vi "temp_till_try_and_error.vi"(6 "Timeout (10000 ms)":u32=10000, 8 "error in (no error)":errorcluster, 9 "Points":i32=250, 10 "Source Channel (0: Channel 1)":i32(ring) items=["Channel 1"=0, "Channel 2"=1, "Channel 3"=2, "Channel 4"=3, "Waveform Memory 1"=5, "Waveform Memory 2"=6, "Serial Bus 1"=7, "Serial Bus 2"=8, "Digital Bus Low"=9, "Digital Bus High "=10, "Digital Bus 1"=11, "Digital Bus 2"=12, "Function 1"=32, "Function 2"=33, "Function 3"=34, "Function 4"=35, "Math 1"=36, "Math 2"=37, "Math 3"=38, "Math 4"=39], 11 "VISA resource name":refnum<visa-resource-name>) -> (0 "error out":errorcluster, 2 "Waveform Data":waveform(dbl)[](graph), 3 "VISA resource name out":refnum<visa-resource-name>)   [LabVIEW 2016]
uses:
  <instrlib>/Agilent 2000 3000 X-Series/Agilent 2000 3000 X-Series.lvlib
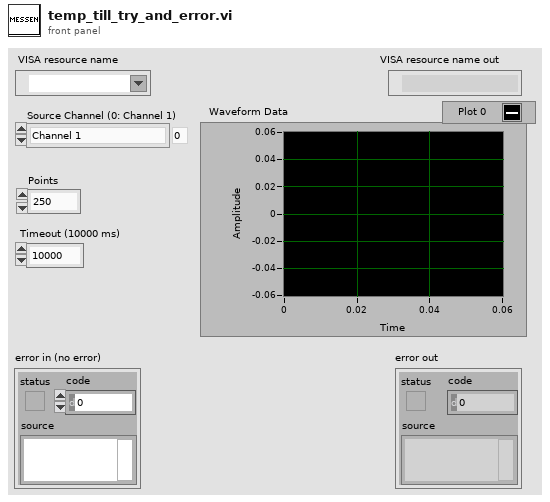
[diagram p1: front panel]
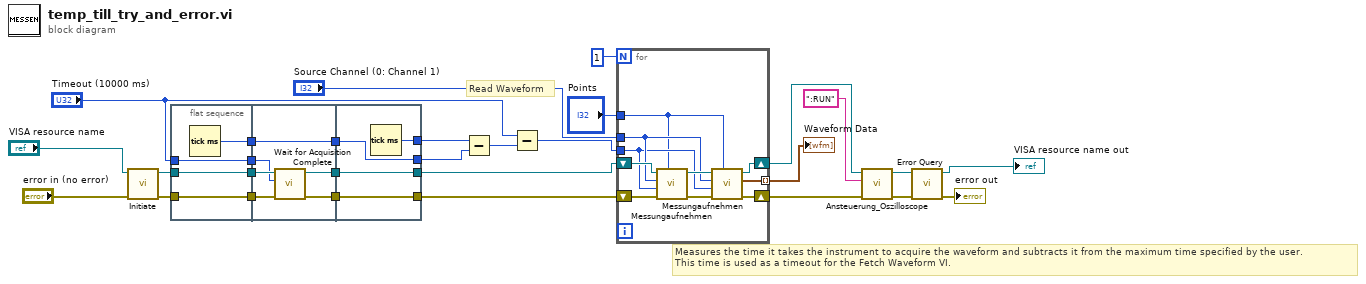
[diagram p0: block diagram]
diagram:
  # "Measures the time it takes the instrument to acquire the waveform and subtracts it from the maximum time specified by the user.\nThis time is used as a timeout for the Fetch Waveform VI."
  # "Read Waveform"
  n1 = call <instrlib>:"Initiate.vi"("error in (no error)"="error in (no error)", "VISA resource name"="VISA resource name") -> ("error out"=w17:errorcluster, "VISA resource name out"=w18:refnum<visa-resource-name>)  [unwired: 8 out]
  n2 = flat-sequence {
    tunnel: w18 -> [w32]
    tunnel: [w32] -> w29
    tunnel: w17 -> [w31]
    tunnel: [w31] -> w28
    tunnel: "Timeout (10000 ms)" -> [w30]
    tunnel: [w30] -> w27
    tunnel: [w33] -> w26
    tunnel: w29 -> [w39]
    tunnel: [w37] -> w25
    tunnel: w28 -> [w38]
    tunnel: [w36] -> w24
    tunnel: w27 -> [w35]
    tunnel: w26 -> [w34]
    tunnel: [w34] -> w23
    tunnel: [w42] -> w11
    tunnel: w25 -> [w42]
    tunnel: [w41] -> w10
    tunnel: w24 -> [w41]
    tunnel: [w40] -> w22
    tunnel: w23 -> [w40]
    tunnel: [w43] -> w21
    frame #0 {
      n3 = Tick Count (ms)() -> (millisecond timer value=w33:u32)
    }
    frame #1 {
      n4 = call <instrlib>:"Wait for Acquisition Complete.vi"("error in (no error)"=w38, "Maximum Time (10000)"=w35, "VISA resource name"=w39) -> ("error out"=w36:errorcluster, "VISA resource name out"=w37:refnum<visa-resource-name>)  [unwired: 7 out]
    }
    frame #2 {
      n5 = Tick Count (ms)() -> (millisecond timer value=w43:u32)
    }
  }
  n6 = Subtract(x=w21, y=w22) -> (x-y=w13:u32)
  n7 = Subtract(x="Timeout (10000 ms)", y=w13) -> (x-y=w9:u32)
  n8 = for {
    N: 1 -> [_]
    tunnel: "Source Channel (0: Channel 1)" -> [w46]
    tunnel: w9 -> [w45]
    tunnel: "Points" -> [w44]
    shift-right: [w49] -> w8
    shift-left: w11 -> [w53]
    shift-right: [w48] -> w7
    shift-left: w10 -> [w52]
    tunnel: [w47] -> w1 mode=indexing
    n9 = call "Messungaufnehmen.vi"("Points"=w44, "error in (no error)"=w52, "Timeout (10000)"=w45, "Source Channel (0: Channel 1)"=w46, "VISA Name OZ in(OZ)"=w53) -> ("error out"=w51:errorcluster, "VISA resource name out"=w50:refnum<visa-resource-name>)  [unwired: 4 in, 1 out]
    n10 = call "Messungaufnehmen.vi"("Points"=w44, "error in (no error)"=w51, "Timeout (10000)"=w45, "Source Channel (0: Channel 1)"=w46, "VISA Name OZ in(OZ)"=w50) -> ("error out"=w48:errorcluster, "Waveform Data"=w47:waveform(dbl), "VISA resource name out"=w49:refnum<visa-resource-name>)  [unwired: 4 in]
  }
  "Waveform Data" <- w1
  n11 = call "Ansteuerung_Oszilloscope.vi"("Error_in"=w7, "Eingangs-String"=":RUN", "VISA Name OZ in(OZ)"=w8) -> ("Error_out"=w5:errorcluster, "VISA Name OZ out"=w6:refnum<visa-resource-name>)  [unwired: 6 in, 1 out]
  n12 = call <instrlib>:"Error Query.vi"("error in (no error)"=w5, "VISA resource name"=w6) -> ("error out"=→"error out":errorcluster, "VISA resource name out"=→"VISA resource name out":refnum<visa-resource-name>)  [unwired: 8 out]
